vi "G# - CreatingAndDestroyingObjects.vi"() -> ()   [LabVIEW 2017]
doc: "This example will show how to create and destroy an object.\nThe classes are created with different templates, but with the exact same methods setting both attributes according to controls.\n\nNotice the difference in how attributes are modified, the value will be set to 2 for both attribures.\n\nThe G#Template performance is better than the G#BaseTemplateG3 when using the Data Value Reference structure.\n\nBy using the G# Debugger found in Tools->G# Debugger a text log can be followed showing how the objects were created and destroyed."
uses:
  MyG#G3Templ_class/MyG#G3Templ.lvclass
  MyG#Class_class/MyG#Class.lvclass
  vi.lib/addons/_AddQ/G#Object/G#Object.lvclass
panel:
  in  "Add G#G3Templ attribute with....":dbl=2.0
  in  "Add G# object attribute with....":dbl=2.0
  in  "My G#G3Templ Attribute in":dbl=12.0
  in  "My G# Object Attribute in":dbl=12.0
  in  "error in (no error)":errorcluster
  out "# of objects killed":i32
  out "OK":bool
  out "My G#G3Templ Attribute out":dbl
  out "My G# Object Attribute out":dbl
  out "error out":errorcluster
  # "This example will show how to create and destroy an object.\nThe classes are created with different templates, but with the exact same methods setting both attributes according to controls.\n\nNotice the difference in how attributes are modified, the value will be set to 2 for both attribures.\n\nThe G#Template performance is better than the G#BaseTemplateG3 when using the Data Value Reference structure.\n\nBy using the G# Debugger found in Tools->G# Debugger a text log can be followed showing how the objects were created and destroyed."
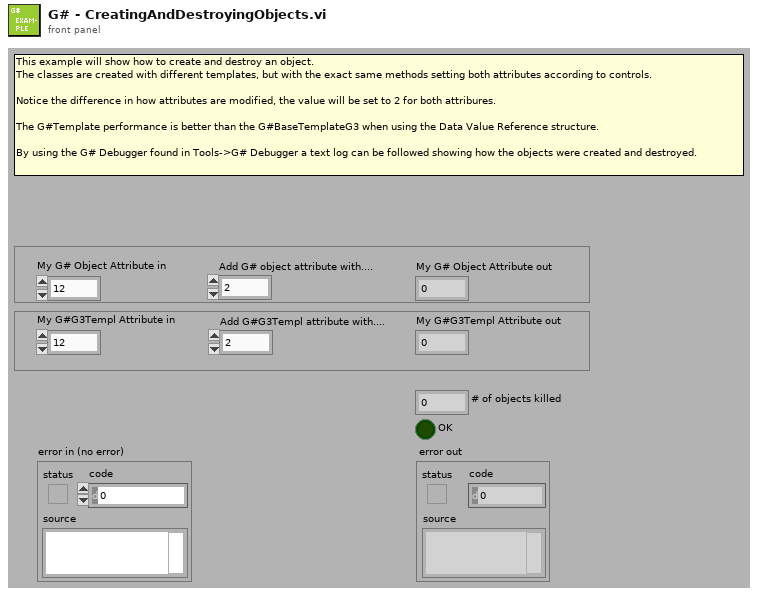
[diagram p1: front panel]
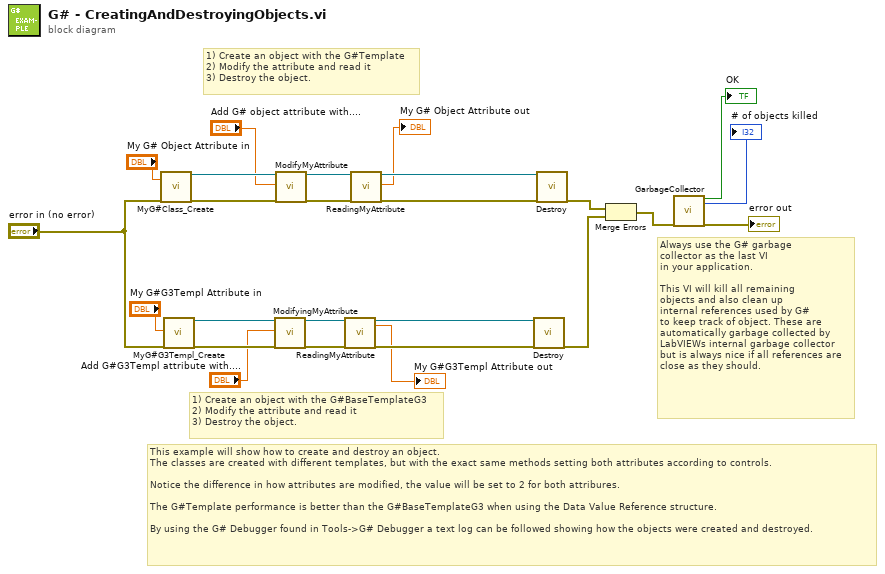
[diagram p0: block diagram]
diagram:
  # "This example will show how to create and destroy an object.\nThe classes are created with different templates, but with the exact same methods setting both attributes according to controls.\n\nNotice the difference in how attributes are modified, the value will be set to 2 for both attribures.\n\nThe G#Template performance is better than the G#BaseTemplateG3 when using the Data Value Reference structure.\n\nBy using the G# Debugger found in Tools->G# Debugger a text log can be followed showing how the objects were created and destroyed."
  # "Always use the G# garbage\ncollector as the last VI\nin your application.\n\nThis VI will kill all remaining\nobjects and also clean up\ninternal references used by G#\nto keep track of object. These are\nautomatically garbage collected by\nLabVIEWs internal garbage collector\nbut is always nice if all references are\nclose as they should."
  # "1) Create an object with the G#BaseTemplateG3\n2) Modify the attribute and read it\n3) Destroy the object."
  # "1) Create an object with the G#Template\n2) Modify the attribute and read it\n3) Destroy the object."
  n1 = call "MyG#Class_Create.vi"("MyAttribute"="My G# Object Attribute in", "error in (no error)"="error in (no error)") -> ("reference out"=w24:refnum<class "MyG#Class.lvclass">, "error out"=w25:errorcluster)  [unwired: 16 in]
  n2 = call "MyG#G3Templ_Create.vi"("MyAttribute"="My G#G3Templ Attribute in", "error in (no error)"="error in (no error)") -> ("reference out"=w14:refnum<class "MyG#G3Templ.lvclass">, "error out"=w19:errorcluster)  [unwired: 16 in]
  n3 = call-dynamic "ModifyingMyAttribute.vi"("reference in"=w14, "increment"="Add G#G3Templ attribute with....", "error in (no error)"=w19) -> ("reference out"=w15:refnum<class "MyG#G3Templ.lvclass">, "error out"=w18:errorcluster)  [unwired: 15 in]
  n4 = call-dynamic "ModifyMyAttribute.vi"("reference in"=w24, "increment"="Add G# object attribute with....", "error in (no error)"=w25) -> ("reference out"=w23:refnum<class "MyG#Class.lvclass">, "error out"=w22:errorcluster)  [unwired: 15 in]
  n5 = call-dynamic "ReadingMyAttribute.vi"("reference in"=w15, "error in (no error)"=w18) -> ("reference out"=w16:refnum<class "MyG#G3Templ.lvclass">, "MyAttribute"=→"My G#G3Templ Attribute out":dbl, "error out"=w17:errorcluster)  [unwired: 15 in]
  n6 = call-dynamic "ReadingMyAttribute.vi"("reference in"=w23, "error in (no error)"=w22) -> ("reference out"=w21:refnum<class "MyG#Class.lvclass">, "MyAttribute"=→"My G# Object Attribute out":dbl, "error out"=w20:errorcluster)  [unwired: 15 in]
  n7 = call-dynamic "Destroy.vi"("reference in"=w16, "error in (no error)"=w17) -> ("error out"=w10:errorcluster)  [unwired: 16 in, 1 out]
  n8 = call-dynamic "Destroy.vi"("reference in"=w21, "error in (no error)"=w20) -> ("error out"=w11:errorcluster)  [unwired: 16 in, 1 out]
  n9 = Merge Errors(w11, w10) -> (w5:errorcluster)
  n10 = call "GarbageCollector.vi"("error in (no error)"=w5) -> ("OK"=→"OK":bool, "# of objects killed"=→"# of objects killed":i32, "error out"=→"error out":errorcluster)  [unwired: 16 in]
